vi "render hold note_blue.vi"(4 "head index":i32, 6 "progress":dbl, 7 "y-center":dbl, 10 "rail":cluster{"note type":string, "position":dbl}[](array[cluster]), 11 "new picture in":picture) -> (3 "new picture out":picture)   [LabVIEW 2023]
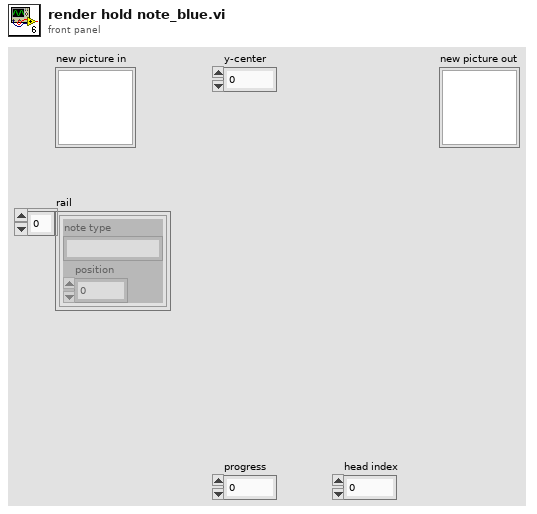
[diagram p1: front panel]
types:
  T1 = cluster{"Width":u16, "Style":enum32{"Solid", "Dash", "Dot", "DashDot", "DashDotDot"}}
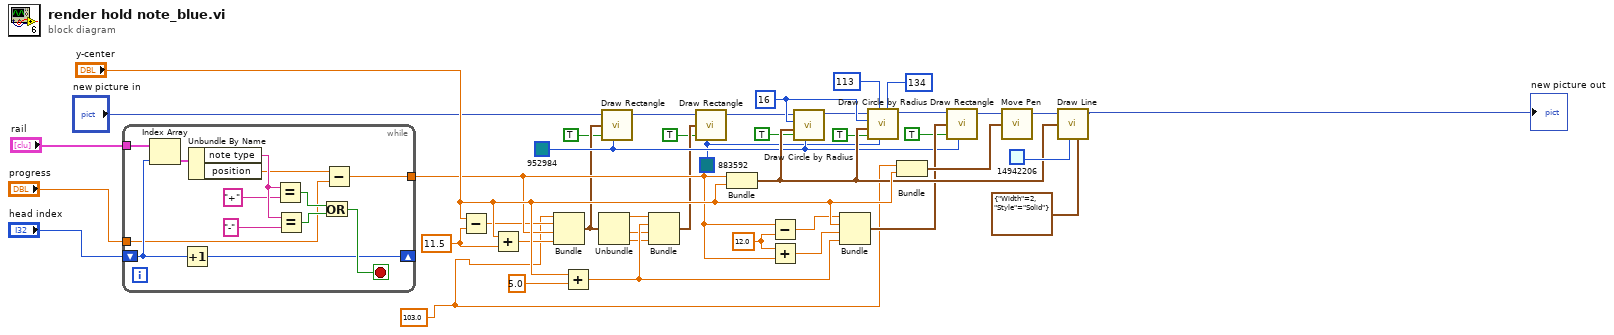
[diagram p0: block diagram]
diagram:
  w1 = 103.0 ("y")
  w30 = 12.0 ("y")
  w22 = u32 883592 ("color(black)")
  w29 = u32 952984 ("color(black)")
  w8 = 11.5 ("y")
  w26 = i16 16 ("radius")
  n1 = while {
    tunnel: "rail" -> [w55]
    shift-right: [w46] -> _
    shift-left: "head index" -> [w47]
    tunnel: "progress" -> [w45]
    tunnel: [w43] -> w31
    stop <- w48 stop-if-true
    n2 = Index Array(array=w55, index=w47) -> (element=w54:cluster{"note type":string, "position":dbl})
    n3 = Increment(x=w47) -> (x+1=w46:i32)
    n4 = Unbundle By Name(w54) -> ("note type"=w51:string, "position"=w44:dbl)
    n5 = Equal?(x=w51, y="+") -> (x = y?=w53:bool)
    n6 = Equal?(x=w51, y="-") -> (x = y?=w52:bool)
    n7 = Or(x=w53, y=w52) -> (x .or. y?=w48:bool)
    n8 = Subtract(x=w44, y=w45) -> (x-y=w43:dbl)
  }
  n9 = Subtract(x="y-center", y=w8) -> (x-y=w7:dbl)
  n10 = Add(x="y-center", y=w8) -> (x+y=w9:dbl)
  n11 = Bundle("y"=w1, w7, w31, w9) -> (w15:cluster{"y":dbl, dbl, dbl, dbl})  [unwired: 1 in]
  n12 = Add(x="y-center", y=5.0) -> (x+y=w34:dbl)
  n13 = Unbundle(w15) -> ("y"=w16:dbl, w17:dbl, w18:dbl)  [unwired: 1 out]
  n14 = call <vilib>:"Draw Rectangle.vi"("picture"="new picture in", "rect"=w15, "fill?(F)"=TRUE, "color(black)"=w29) -> ("new picture"=w12:picture)  [unwired: 5 in]
  n15 = Bundle("y"=w16, w34, w17, w18) -> (w20:cluster{"y":dbl, dbl, dbl, dbl})  [unwired: 1 in]
  n16 = call <vilib>:"Draw Rectangle.vi"("picture"=w12, "rect"=w20, "fill?(F)"=TRUE, "color(black)"=w22) -> ("new picture"=w13:picture)  [unwired: 5 in]
  n17 = Bundle(w31, "y-center"="y-center") -> (w39:cluster{dbl, "y-center":dbl})  [unwired: 1 in]
  n18 = Subtract(x=w31, y=w30) -> (x-y=w32:dbl)
  n19 = Add(x=w30, y=w31) -> (x+y=w33:dbl)
  n20 = call <vilib>:"Draw Circle by Radius.vi"("color(black)"=w29, "fill?(F)"=TRUE, "pixel center"=w39, "radius"=w26, "picture"=w13) -> ("new picture"=w21:picture)  [unwired: 6 in]
  n21 = Bundle(w32, "y-center"="y-center", w33, w34) -> (w35:cluster{dbl, "y-center":dbl, dbl, dbl})  [unwired: 1 in]
  n22 = call <vilib>:"Draw Circle by Radius.vi"("arc size(360)"=i16 134 ("radius"), "color(black)"=w22, "start angle(0)"=i16 113 ("radius"), "fill?(F)"=TRUE, "pixel center"=w39, "radius"=w26, "picture"=w21) -> ("new picture"=w27:picture)  [unwired: 4 in]
  n23 = Bundle("y"=w1, "y-center"="y-center") -> (w37:cluster{"y":dbl, "y-center":dbl})  [unwired: 1 in]
  n24 = call <vilib>:"Draw Rectangle.vi"("picture"=w27, "rect"=w35, "fill?(F)"=TRUE, "color(black)"=w29) -> ("new picture"=w36:picture)  [unwired: 5 in]
  n25 = call <vilib>:"Move Pen.vi"("new position"=w37, "picture"=w36) -> ("new picture"=w38:picture)  [unwired: 3 in]
  n26 = call <vilib>:"Draw Line.vi"("picture"=w38, "end point"=w39, "color(black)"=u32 14942206, "pen"=T1 {"Width"=2, "Style"=enum."Solid"}) -> ("new picture"=→"new picture out":picture)  [unwired: 5 in]
